vi "Check Autostart.vi"(8 "error in (no error)":errorcluster, 11 "Application in":refnum<class "Application.lvclass">) -> (0 "error out":errorcluster, 2 "Start Test":bool, 3 "Application out":refnum<class "Application.lvclass">)   [LabVIEW 2015, in "Application.lvlib" / "Application.lvclass"]
doc: "Used by child classes to perform a check of some physical hardware. If TRUE this will start the test."
uses:
  Application.lvclass
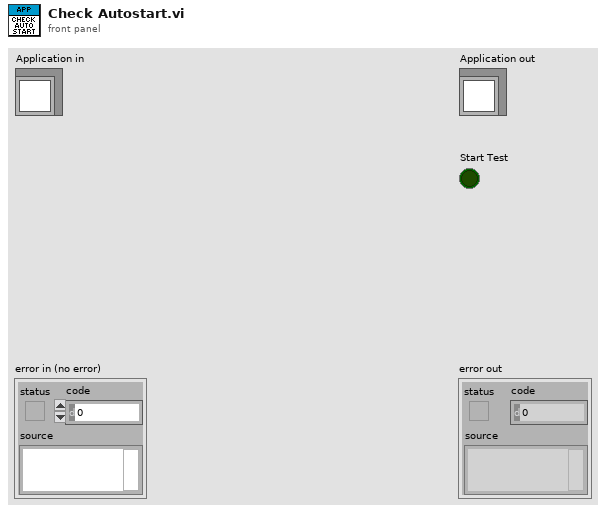
[diagram p1: front panel]
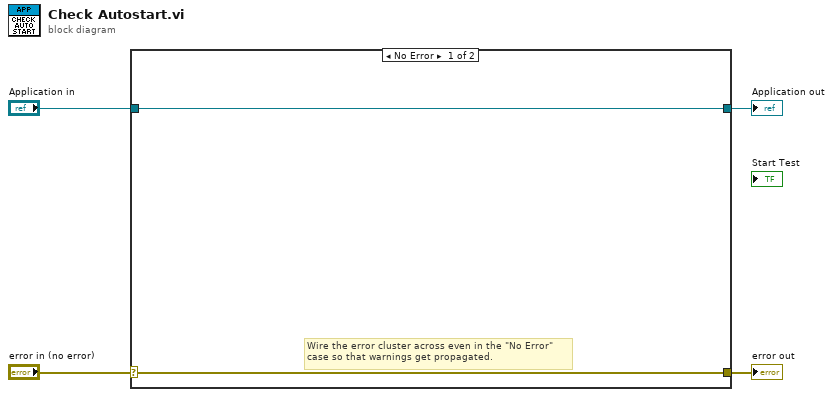
[diagram p0: block diagram]
diagram:
  n1 = case shown="No Error" "error in (no error)" {
    selector: "error in (no error)" -> [w5 w8]
    tunnel: [w5 w8] -> w3
    tunnel: [w6 w7] -> w1
    tunnel: "Application in" -> [w6 w7]
    frame No Error {
      # "Wire the error cluster across even in the \"No Error\"\ncase so that warnings get propagated."
    }
    frame Error {
    }
  }
  "error out" <- w3
  "Application out" <- w1
